vi "PlateReaderGlobal.vi"() -> ()   [LabVIEW 2014]
uses:
  EventHandleCommandCompletedData.ctl
  EventHandleInstrumentStatusChangedData.ctl
  EventHandleErrorReportData.ctl
panel:
  out "Stop":bool
  out "Mark Read Stop Time":timestamp
  out "Mark Read Start Time":timestamp
  out "Change from Busy Time":timestamp
  out "Change to Busy Time":timestamp
  out "ErrorReportQueue":refnum<queue>
  out "CommandCompleteQueue":refnum<queue>
  out "Last ErrorReport Cluster":T1
  out "Last InstrumentStatusChanged Cluster":T2
  out "Last CommandCompleted Cluster":T3
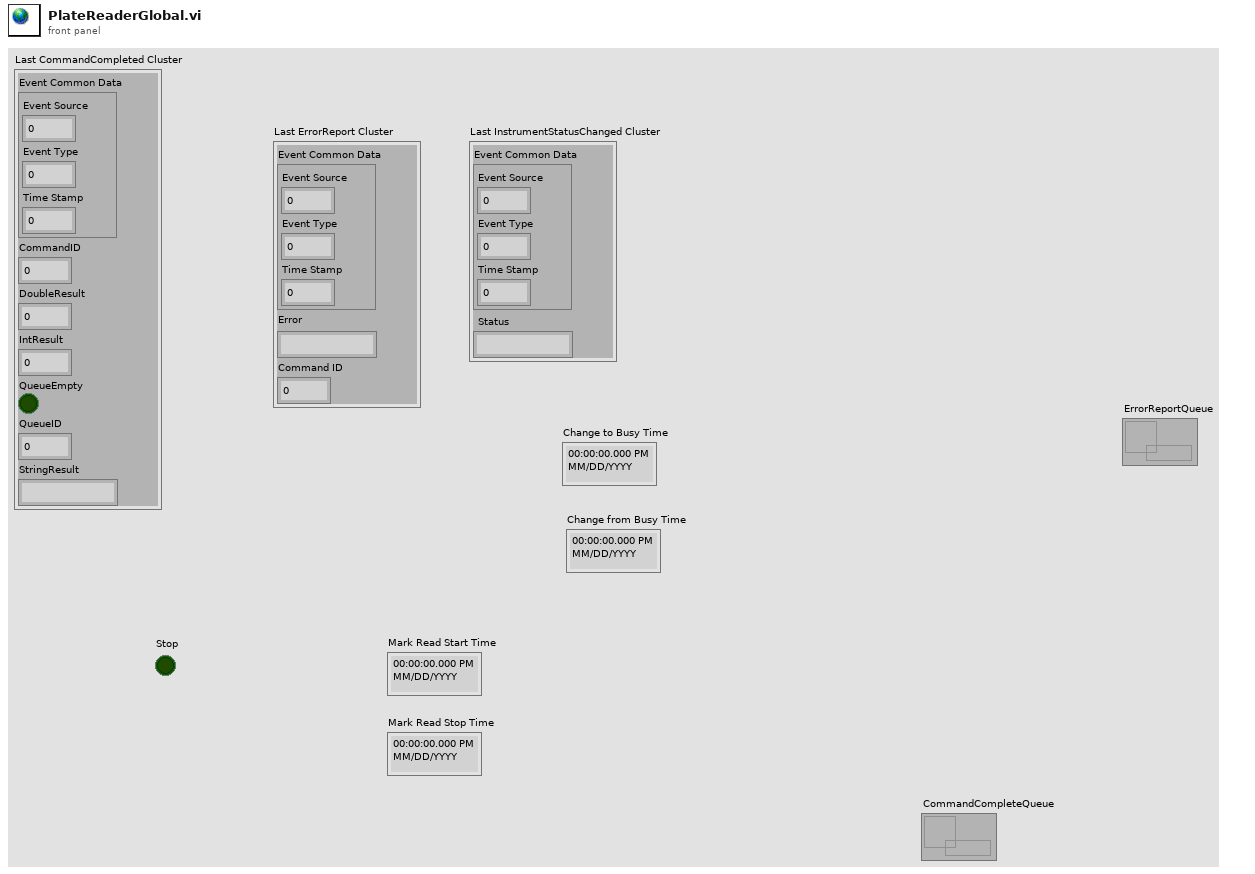
[diagram p1: front panel]
types:
  T1 = typedef "EventHandleErrorReportData.ctl" = cluster{"Event Common Data":cluster{"Event Source":i32, "Event Type":u32, "Time Stamp":u32}, "Error":string, "Command ID":i32}
  T2 = typedef "EventHandleInstrumentStatusChangedData.ctl" = cluster{"Event Common Data":cluster{"Event Source":i32, "Event Type":u32, "Time Stamp":u32}, "Status":string}
  T3 = typedef "EventHandleCommandCompletedData.ctl" = cluster{"Event Common Data":cluster{"Event Source":i32, "Event Type":u32, "Time Stamp":u32}, "CommandID":i32, "DoubleResult":dbl, "IntResult":i32, "QueueEmpty":bool, "QueueID":i32, "StringResult":string}
diagram:
